vi "Skyline_ReadWritePoly.vi"   [LabVIEW 2016]
uses:
  Systemlink Tag.xctl
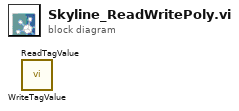
[diagram p0: block diagram]
diagram:
  n1 = call "WriteTagValue.vi"() -> ()  [unwired: 12 in]
  n2 = call "ReadTagValue.vi"() -> ()  [unwired: 10 in, 2 out]
